vi "SaveRefsPilMOT.vi"(6 "Numéro d'axe":i32, 7 "error in":errorcluster, 8 "Référence à enregistrer":i32, 9 "Num de Ref à enregistrer":i32, 10 "file path (use dialog)":path) -> (0 "error out":errorcluster)   [LabVIEW 2013]
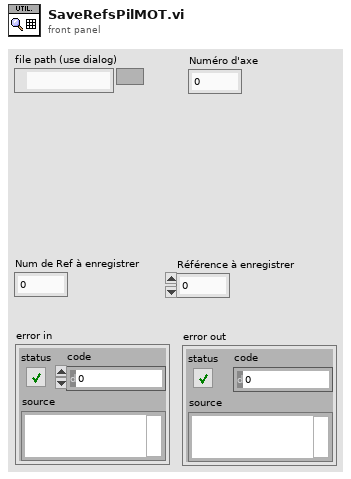
[diagram p1: front panel]
types:
  T1 = enum16{"open", "replace", "create", "open or create", "replace or create", "replace or create with confirmation"}
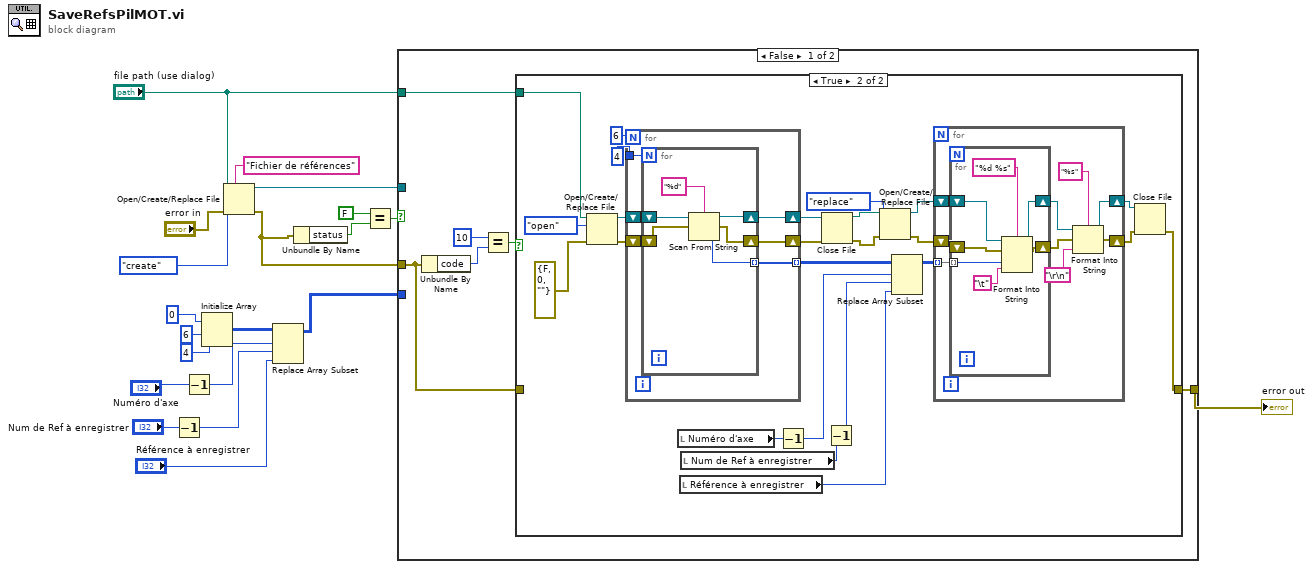
[diagram p0: block diagram]
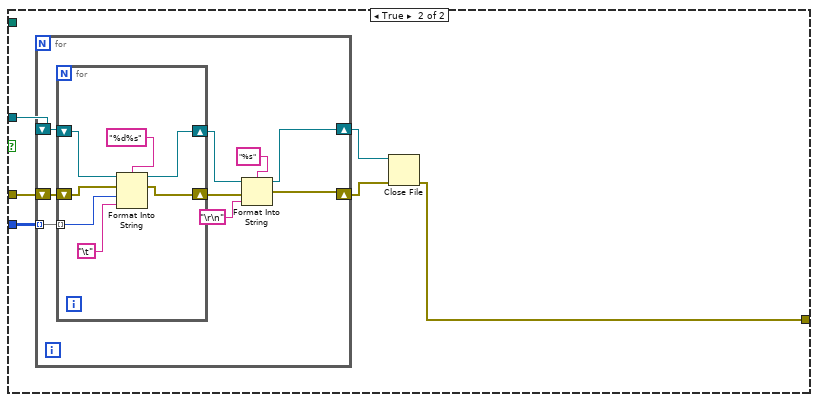
[diagram p3: hidden frame]
diagram:
  n1 = Decrement(x="Num de Ref à enregistrer") -> (x-1=w2:i32)
  n2 = Decrement(x="Numéro d'axe") -> (x-1=w3:i32)
  n3 = Initialize Array(0 ("Référence à enregistrer"), 6 ("dimension size"), 4 ("dimension size")) -> (w8:i32[][])
  n4 = Open/Create/Replace File(file path (use dialog)="file path (use dialog)", error in="error in", prompt="Fichier de références", operation (0:open)=T1."create") -> (refnum out=w18:refnum<file>, error out=w15:errorcluster)  [unwired: 2 in, 1 out]
  n5 = Replace Array Subset(array=w8, new element="Référence à enregistrer", index (row)=w3, index (col)=w2) -> (w4:i32[][])
  n6 = Unbundle By Name(w15) -> ("status"=w14:bool)
  n7 = Equal?(x=FALSE, y=w14) -> (x = y?=w13:bool)
  n8 = case shown="False" w13 {
    tunnel: w4 -> [_ w85]
    tunnel: w15 -> [w21 w84]
    tunnel: w18 -> [_ w83]
    tunnel: [w22 w80] -> w17
    tunnel: "file path (use dialog)" -> [w23 _]
    frame False {
      n9 = Unbundle By Name(w21) -> ("code"=w26:i32)
      n10 = Equal?(x=10, y=w26) -> (x = y?=w24:bool)
      n11 = case shown="True" w24 {
        tunnel: w23 -> [_ w51]
        tunnel: [w27 w38] -> w22
        tunnel: w21 -> [w27 _]
        frame False {
        }
        frame True {
          n12 = Open/Create/Replace File(file path (use dialog)=w51, error in=errorcluster {"status"=FALSE, "code"=0, "source"=""}, operation (0:open)=T1."open") -> (refnum out=w48:refnum<file>, error out=w47:errorcluster)  [unwired: 3 in, 1 out]
          n13 = for {
            N: 6 -> [_]
            tunnel: 4 -> [w71]
            shift-right: [w69] -> w36
            shift-left: w47 -> [w72]
            shift-right: [w70] -> w37
            shift-left: w48 -> [w73]
            tunnel: [w68] -> w44 mode=indexing
            n14 = for {
              N: w71 -> [_]
              shift-right: [w76] -> w69
              shift-left: w72 -> [w78]
              shift-right: [w75] -> w70
              shift-left: w73 -> [w79]
              tunnel: [w74] -> w68 mode=indexing
              n15 = Scan From String("%d" ("format string"), w79, w78) -> (w75:refnum<file>, w76:errorcluster, output 1=w74:i32)  [unwired: 1 in]
            }
          }
          n16 = local read "Numéro d'axe"() -> (w43:i32)
          n17 = local read "Référence à enregistrer"() -> (w41:i32)
          n18 = local read "Num de Ref à enregistrer"() -> (w42:i32)
          n19 = Decrement(x=w43) -> (x-1=w30:i32)
          n20 = Close File(refnum=w37, error in=w36) -> (path=w33:path, error out=w31:errorcluster)
          n21 = Decrement(x=w42) -> (x-1=w29:i32)
          n22 = Open/Create/Replace File(file path (use dialog)=w33, error in=w31, operation (0:open)=T1."replace") -> (refnum out=w34:refnum<file>, error out=w35:errorcluster)  [unwired: 3 in, 1 out]
          n23 = Replace Array Subset(array=w44, new element=w41, index (row)=w30, index (col)=w29) -> (w45:i32[][])
          n24 = for {
            tunnel: w45 -> [w60] mode=indexing
            shift-right: [w52] -> w40
            shift-left: w35 -> [w58]
            shift-right: [w54] -> w39
            shift-left: w34 -> [w59]
            n25 = for {
              tunnel: w60 -> [w67] mode=indexing
              shift-right: [w64] -> w56
              shift-left: w58 -> [w65]
              shift-right: [w62] -> w55
              shift-left: w59 -> [w66]
              n26 = Format Into String(format string="%d %s", initial string=w66, error in=w65, w67, "\t") -> (resulting string=w62:refnum<file>, error out=w64:errorcluster)
            }
            n27 = Format Into String(format string="%s", initial string=w55, error in=w56, "\r\n") -> (resulting string=w54:refnum<file>, error out=w52:errorcluster)
          }
          n28 = Close File(refnum=w39, error in=w40) -> (error out=w38:errorcluster)  [unwired: 1 out]
        }
      }
    }
    frame True {
      n29 = for {
        tunnel: w85 -> [w94] mode=indexing
        shift-right: [w87] -> w81
        shift-left: w84 -> [w93]
        shift-right: [w88] -> w82
        shift-left: w83 -> [w91]
        n30 = for {
          tunnel: w94 -> [w100] mode=indexing
          shift-right: [w97] -> w92
          shift-left: w93 -> [w98]
          shift-right: [w95] -> w90
          shift-left: w91 -> [w96]
          n31 = Format Into String(format string="%d%s", initial string=w96, error in=w98, w100, "\t") -> (resulting string=w95:refnum<file>, error out=w97:errorcluster)
        }
        n32 = Format Into String(format string="%s", initial string=w90, error in=w92, "\r\n") -> (resulting string=w88:refnum<file>, error out=w87:errorcluster)
      }
      n33 = Close File(refnum=w82, error in=w81) -> (error out=w80:errorcluster)  [unwired: 1 out]
    }
  }
  "error out" <- w17
